vi "saveDataNodeBegin.vi"(8 "error in (no error)":errorcluster, 9 "indent":i32, 10 "XML Refnum in":refnum<file>, 11 "xceDataNode in":refnum<class "xceDataNode.lvclass">) -> (0 "error out":errorcluster, 2 "XML Refnum out":refnum<file>, 3 "xceDataNode out":refnum<class "xceDataNode.lvclass">)   [LabVIEW 2013, in "xceDataNode.lvclass"]
doc: "Begins the process of saving a xceData Node to an XML formatted file."
uses:
  xceDataNode.lvclass
  xceDataNode.lvclass/xceDataNode.ctl
  xceNode/xceNode.lvclass
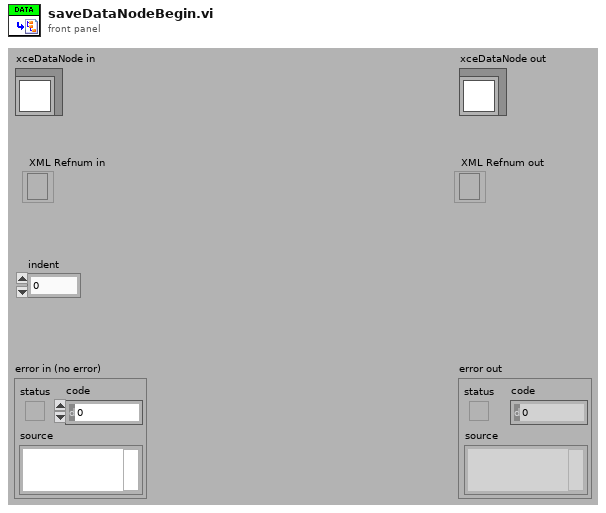
[diagram p1: front panel]
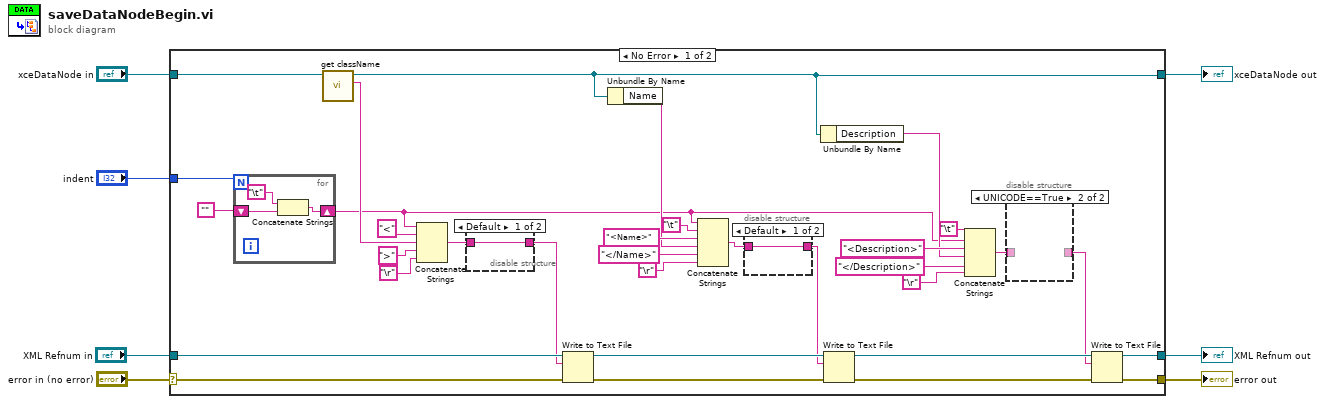
[diagram p0: block diagram]
diagram:
  n1 = case shown="No Error" "error in (no error)" {
    selector: "error in (no error)" -> [w33 w49]
    tunnel: [w9 w49] -> w6
    tunnel: [w10 w48] -> w4
    tunnel: "xceDataNode in" -> [w39 w48]
    tunnel: "indent" -> [w12 _]
    tunnel: "XML Refnum in" -> [w32 w47]
    tunnel: [w8 w47] -> w1
    frame No Error {
      n2 = for {
        N: w12 -> [_]
        shift-right: [w46] -> w11
        shift-left: "" -> [w45]
        n3 = Concatenate Strings("\t", w45) -> (w46:string)
      }
      n4 = call "get className.vi"("xceNode in"=w39) -> ("Class name"=w37:string, "xceNode out"=w10:refnum<class "xceDataNode.lvclass">)  [unwired: 8 in, 1 out]
      n5 = Concatenate Strings(w11, "<", w37, ">", "\r") -> (w34:string)
      n6 = disable-structure shown="Default" {
        disable-tunnel: w34 -> [w43 _]
        disable-tunnel: [w43 _] -> w31
        frame condition #0 (active) {
        }
        frame condition #1 {
        }
      }
      n7 = Write to Text File(file (use dialog)=w32, text=w31, error in=w33) -> (refnum out=w25:refnum<file>, error out=w23:errorcluster)  [unwired: 1 in, 1 out]
      n8 = Unbundle By Name(w10) -> ("Name"=w29:string)
      n9 = Concatenate Strings(w11, "\t", "<Name>", w29, "</Name>" ("string"), "\r") -> (w26:string)
      n10 = disable-structure shown="Default" {
        disable-tunnel: w26 -> [w42 _]
        disable-tunnel: [w42 _] -> w24
        frame condition #0 (active) {
        }
        frame condition #1 {
        }
      }
      n11 = Unbundle By Name(w10) -> ("Description"=w21:string)
      n12 = Write to Text File(file (use dialog)=w25, text=w24, error in=w23) -> (refnum out=w15:refnum<file>, error out=w14:errorcluster)  [unwired: 1 in, 1 out]
      n13 = Concatenate Strings("\t", w11, "<Description>" ("string"), w21, "</Description>" ("string"), "\r") -> (w16:string)
      n14 = disable-structure shown="UNICODE==True" {
        disable-tunnel: w16 -> [w41 _]
        disable-tunnel: [w41 _] -> w13
        frame condition #0 (active) {
        }
        frame condition #1 {
        }
      }
      n15 = Write to Text File(file (use dialog)=w15, text=w13, error in=w14) -> (refnum out=w8:refnum<file>, error out=w9:errorcluster)  [unwired: 1 in, 1 out]
    }
    frame Error {
    }
  }
  "error out" <- w6
  "xceDataNode out" <- w4
  "XML Refnum out" <- w1
